vi "TrajConstraint_GetMinMaxAccel.vi"(7 "TrajjectoryConstraintType":T5, 8 "Velocity":dbl, 9 "Curvature":dbl, 10 "Pose":T2={"TRANSLATION"={"X"=0.0, "Y"=0.0}, "ROTATION"={"VALUE"=0.0, "COS"=1.0, "SIN"=0.0}} {"ROTATION"."SIN" format="%13.4f"; "ROTATION"."COS" format="%13.4f"; "ROTATION"."VALUE" format="%13.4f"; "TRANSLATION"."Y" format="%14.3f"; "TRANSLATION"."X" format="%14.3f"}, 11 "Trajectory Constraint":variant) -> (3 "Min Max Accel":T1)   [LabVIEW 2019, in "Trajectory_Library.lvlib"]
doc: "Adds and enables a centripital acceleration constraint to ensure that the rotating capability of the robot is not exceeded.\n\nParameters:\n - MaxCentAccel - The maximum centripetal acceleration (meters/sec^2)\n - InTrajectoryConfig - The trajectory configuration data structure\n\nReturns:\n - OutTrajectoryConfig - Modified trajectory configuration data structure\n modified to conain them."
uses:
  Trajectory_Library.lvlib
  Enum/TRAJ_CONSTRAINT_TYPES_ENUM.ctl
  TypeDef/POSE2D.ctl
  TypeDef/TRANSLATION2D.ctl
  TypeDef/ROTATION2D.ctl
  TypeDef/TRAJ_CONSTRAINT_MINMAX.ctl
  TypeDef/TRAJ_CONSTRAINT_DIIF_DRIVE_KINEMATICS.ctl
  TypeDef/DIFF_DRIVE_KINEMATICS.ctl
  TypeDef/TRAJ_CONSTRAINT_DIIF_DRIVE_VOLTAGE.ctl
  TypeDef/SIMPLE_MOTOR_FF.ctl
  TypeDef/TRAJ_CONSTRAINT_CENTRIPETAL_ACCEL.ctl
  TypeDef/TRAJ_CONSTRAINT_MECA_DRIVE_KINEMATICS.ctl
  TypeDef/MECA_DRIVE_KINEMATICS.ctl
  <vilib>/Analysis/Matrix/Datatypes/RealMatrix.ctl
  TypeDef/TRAJ_CONSTRAINT_SWERVE_DRIVE_KINEMATICS.ctl
  TypeDef/SWERVE_DRIVE_KINEMATICS.ctl
  TypeDef/TRAJ_CONSTRAINT_MAX_VELOCITY.ctl
  <vilib>/Analysis/Matrix/NI_Matrix.lvlib
panel:
  out "error out":errorcluster
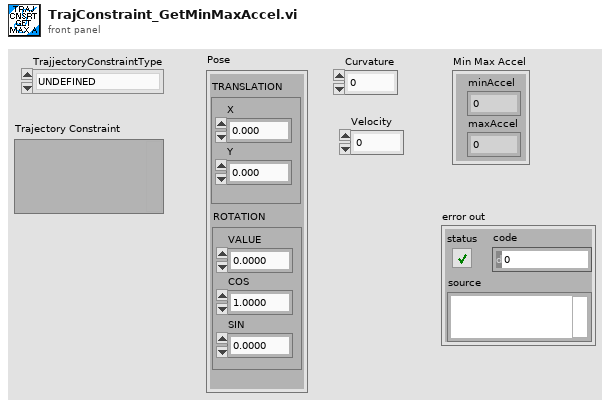
[diagram p1: front panel]
types:
  T1 = typedef "Trajectory_Library.lvlib/TRAJ_CONSTRAINT_MINMAX.ctl" = cluster{"minAccel":dbl, "maxAccel":dbl}
  T2 = typedef "Trajectory_Library.lvlib/POSE2D.ctl" = cluster{"TRANSLATION":T3, "ROTATION":T4}
  T3 = typedef "Trajectory_Library.lvlib/TRANSLATION2D.ctl" = cluster{"X":dbl, "Y":dbl}
  T4 = typedef "Trajectory_Library.lvlib/ROTATION2D.ctl" = cluster{"VALUE":dbl, "COS":dbl, "SIN":dbl}
  T5 = typedef "Trajectory_Library.lvlib/TRAJ_CONSTRAINT_TYPES_ENUM.ctl" = enum16{"UNDEFINED", "DIFF DRIVE KINEMATICS", "DIFF DRIVE VOLTAGE", "CENTRIPITAL ACCEL", "MECA DRIVE KINEMATICS", "SWERVE DRIVE KINEMATICS", "MAXIMUM VELOCITY", "ELLIPTICAL REGION", "RECTANGULAR REGION"}
  T6 = typedef "Trajectory_Library.lvlib/TRAJ_CONSTRAINT_DIIF_DRIVE_KINEMATICS.ctl" = cluster{"Max Speed (M/S)":dbl, "DIFF_DRIVE_KINEMATICS":T7, "Max Accel (M/S2)":dbl}
  T7 = typedef "Trajectory_Library.lvlib/DIFF_DRIVE_KINEMATICS.ctl" = cluster{"TrackWidth_Meters":dbl}
  T8 = typedef "Trajectory_Library.lvlib/TRAJ_CONSTRAINT_DIIF_DRIVE_VOLTAGE.ctl" = cluster{"Max Voltage":dbl, "DIFF_DRIVE_KINEMATICS":T7, "SIMPLE_MOTOR_FF":T9}
  T9 = typedef "Trajectory_Library.lvlib/SIMPLE_MOTOR_FF.ctl" = cluster{"Ks":dbl, "Kv":dbl, "Ka":dbl}
  T10 = typedef "Trajectory_Library.lvlib/TRAJ_CONSTRAINT_CENTRIPETAL_ACCEL.ctl" = cluster{"Max Cent Accel":dbl}
  T11 = typedef "Trajectory_Library.lvlib/TRAJ_CONSTRAINT_MECA_DRIVE_KINEMATICS.ctl" = cluster{"Max Speed (M/S)":dbl, "MECA_DRIVE_KINEMATICS":T12}
  T12 = typedef "Trajectory_Library.lvlib/MECA_DRIVE_KINEMATICS.ctl" = cluster{"FrontLeft":T3, "FrontRight":T3, "RearLeft":T3, "RearRight":T3, "InverseKinematics":T13, "ForwardKinematics":T13, "PrevCoR":T3}
  T13 = typedef "NI_Matrix.lvlib/RealMatrix.ctl" = dbl[][]
  T14 = typedef "Trajectory_Library.lvlib/TRAJ_CONSTRAINT_SWERVE_DRIVE_KINEMATICS.ctl" = cluster{"Max Speed (M/S)":dbl, "SwerveKinematics":T15}
  T15 = typedef "Trajectory_Library.lvlib/SWERVE_DRIVE_KINEMATICS.ctl" = cluster{"NumModules":i32, "InverseKinematics":T13, "ForwardKinematics":T13, "Modules":T3[], "PrevCoR":T3}
  T16 = typedef "Trajectory_Library.lvlib/TRAJ_CONSTRAINT_MAX_VELOCITY.ctl" = cluster{"Max Velocity":dbl, "IM UNIQUE":bool}
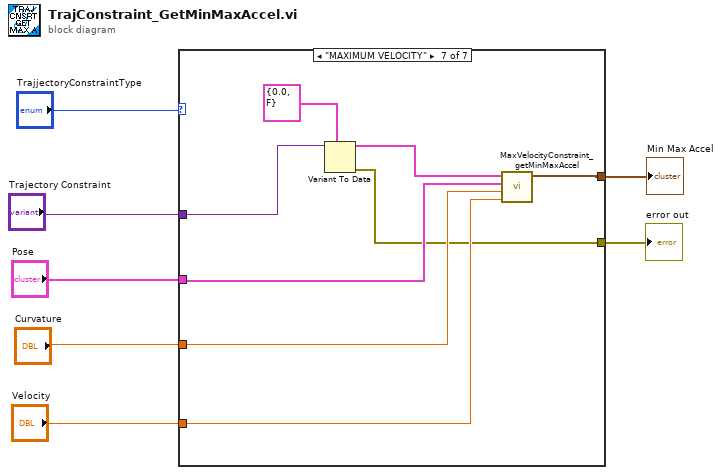
[diagram p0: block diagram]
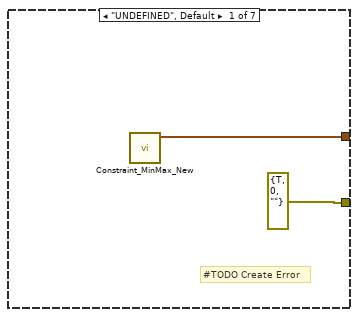
[diagram p2: hidden frame]
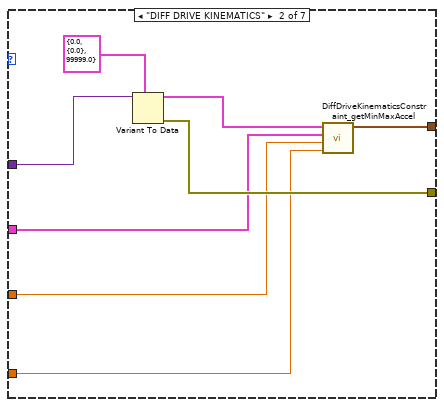
[diagram p3: hidden frame]
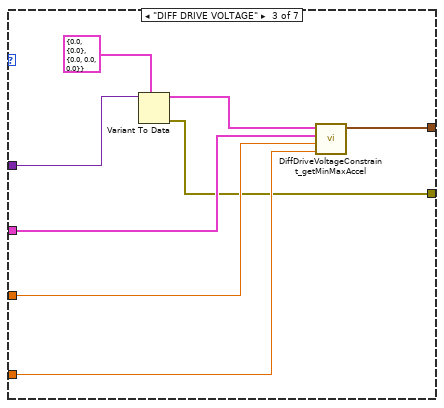
[diagram p4: hidden frame]
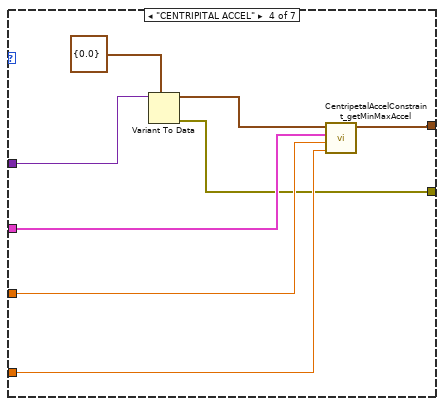
[diagram p5: hidden frame]
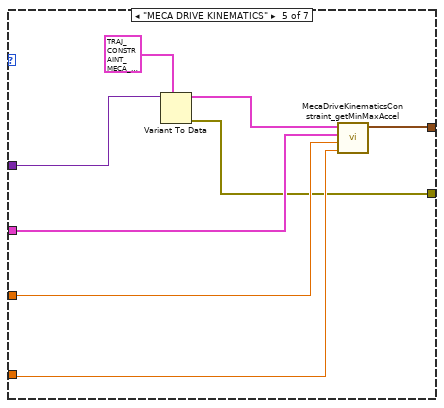
[diagram p6: hidden frame]
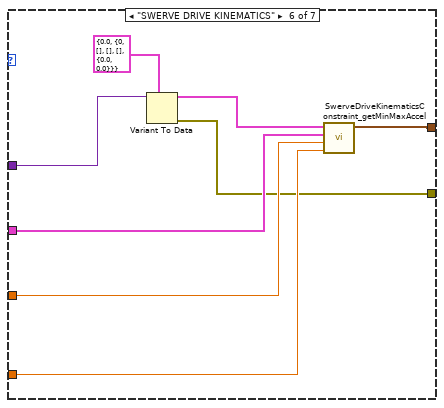
[diagram p7: hidden frame]
diagram:
  n1 = case shown="\"MAXIMUM VELOCITY\"" "TrajjectoryConstraintType" {
    tunnel: [w8 w13 w18 w26 w34 w42 w55] -> w6
    tunnel: "Trajectory Constraint" -> [_ w16 w20 w27 w35 w43 w51]
    tunnel: [errorcluster {"status"=TRUE, "code"=0, "source"=""} ("error out") w15 w19 w28 w36 w44 w50] -> w4
    tunnel: "Pose" -> [_ w12 w23 w31 w39 w47 w54]
    tunnel: "Curvature" -> [_ w11 w22 w30 w38 w46 w53]
    tunnel: "Velocity" -> [_ w10 w21 w29 w37 w45 w52]
    frame "UNDEFINED", Default {
      # "#TODO Create Error"
      n2 = call "Constraint_MinMax_New.vi"() -> ("TRAJ_CONSTAINT_MIN_MAX"=w8:T1)  [unwired: 11 in]
    }
    frame "DIFF DRIVE KINEMATICS" {
      n3 = Variant To Data(type=T6 {"Max Speed (M/S)"=0.0, "DIFF_DRIVE_KINEMATICS"={"TrackWidth_Meters"=0.0}, "Max Accel (M/S2)"=99999.0} ("DIFF_DRIVE_KINE_CONSTRAINT"), Variant=w16) -> (data=w14:T6, error out=w15:errorcluster)  [unwired: 1 in]
      n4 = call "DiffDriveKinematicsConstraint_getMinMaxAccel.vi"("Velocity_M/S"=w10, "Curvature"=w11, "statePose"=w12, "DIFF_DRIVE_KINE_CONSTRAINT"=w14) -> ("TRAJ_CONSTAINT_MIN_MAX"=w13:T1)  [unwired: 7 in]
    }
    frame "DIFF DRIVE VOLTAGE" {
      n5 = Variant To Data(type=T8 {"Max Voltage"=0.0, "DIFF_DRIVE_KINEMATICS"={"TrackWidth_Meters"=0.0}, "SIMPLE_MOTOR_FF"={"Ks"=0.0, "Kv"=0.0, "Ka"=0.0}} ("DIFF_DRIVE_VOLTAGE_CONSTRAINT"), Variant=w20) -> (data=w24:T8, error out=w19:errorcluster)  [unwired: 1 in]
      n6 = call "DiffDriveVoltageConstraint_getMinMaxAccel.vi"("Velocity"=w21, "Curvature"=w22, "statePose"=w23, "DIFF_DRIVE_VOLTAGE_CONSTRAINT"=w24) -> ("TRAJ_CONSTAINT_MIN_MAX"=w18:T1)  [unwired: 7 in]
    }
    frame "CENTRIPITAL ACCEL" {
      n7 = Variant To Data(type=T10 {"Max Cent Accel"=0.0} ("CENTRIPETAL_ACCEL_CONSTRAINT"), Variant=w27) -> (data=w32:T10, error out=w28:errorcluster)  [unwired: 1 in]
      n8 = call "CentripetalAccelConstraint_getMinMaxAccel.vi"("maxVelocity"=w29, "Curvature"=w30, "statePose"=w31, "CENTRIPETAL_ACCEL_CONSTRAINT"=w32) -> ("TRAJ_CONSTAINT_MIN_MAX"=w26:T1)  [unwired: 7 in]
    }
    frame "MECA DRIVE KINEMATICS" {
      n9 = Variant To Data(type=T11 {"Max Speed (M/S)"=0.0, "MECA_DRIVE_KINEMATICS"={"FrontLeft"={"X"=0.0, "Y"=0.0}, "FrontRight"={"X"=0.0, "Y"=0.0}, "RearLeft"={"X"=0.0, "Y"=0.0}, "RearRight"={"X"=0.0, "Y"=0.0}, "InverseKinematics"=[[0.0, 1.0, -1.0, 0.0], [0.0, 1.0, 1.0, 0.0], [0.0, 1.0, 1.0, 0.0], [0.0, 1.0, -1.0, 0.0]], "ForwardKinematics"=[[0.0, 1.0, -1.0, 0.0], [0.0, 1.0, 1.0, 0.0], [0.0, 1.0, 1.0, 0.0], [0.0, 1.0, -1.0, 0.0]], "PrevCoR"={"X"=0.0, "Y"=0.0}}} ("MECANUM_DRIVE_KINE_CONSTRAINT"), Variant=w35) -> (data=w40:T11, error out=w36:errorcluster)  [unwired: 1 in]
      n10 = call "MecaDriveKinematicsConstraint_getMinMaxAccel.vi"("maxVelocity"=w37, "Curvature"=w38, "statePose"=w39, "MECANUM_DRIVE_KINE_CONSTRAINT"=w40) -> ("TRAJ_CONSTAINT_MIN_MAX"=w34:T1)  [unwired: 7 in]
    }
    frame "SWERVE DRIVE KINEMATICS" {
      n11 = Variant To Data(type=T14 {"Max Speed (M/S)"=0.0, "SwerveKinematics"={"NumModules"=0, "InverseKinematics"=[], "ForwardKinematics"=[], "Modules"=[], "PrevCoR"={"X"=0.0, "Y"=0.0}}} ("SWERVE_DRIVE_KINE_CONSTRAINT"), Variant=w43) -> (data=w48:T14, error out=w44:errorcluster)  [unwired: 1 in]
      n12 = call "SwerveDriveKinematicsConstraint_getMinMaxAccel.vi"("maxVelocity"=w45, "Curvature"=w46, "statePose"=w47, "SWERVE_DRIVE_KINE_CONSTRAINT"=w48) -> ("TRAJ_CONSTAINT_MIN_MAX"=w42:T1)  [unwired: 7 in]
    }
    frame "MAXIMUM VELOCITY" {
      n13 = Variant To Data(type=T16 {"Max Velocity"=0.0, "IM UNIQUE"=FALSE} ("MAX_VELOCITY_CONSTRAINT"), Variant=w51) -> (data=w56:T16, error out=w50:errorcluster)  [unwired: 1 in]
      n14 = call "MaxVelocityConstraint_getMinMaxAccel.vi"("maxVelocity"=w52, "Curvature"=w53, "statePose"=w54, "MAX_VELOCITY_CONSTRAINT"=w56) -> ("TRAJ_CONSTAINT_MIN_MAX"=w55:T1)  [unwired: 7 in]
    }
  }
  "Min Max Accel" <- w6
  "error out" <- w4
